vi "Populate Variant Database.vi"(8 "Error In":errorcluster, 10 "Data":string) -> (0 "Error Out":errorcluster, 1 "Variant DB":variant)   [LabVIEW 2017, in "Configit.lvlib"]
uses:
  Configit.lvlib
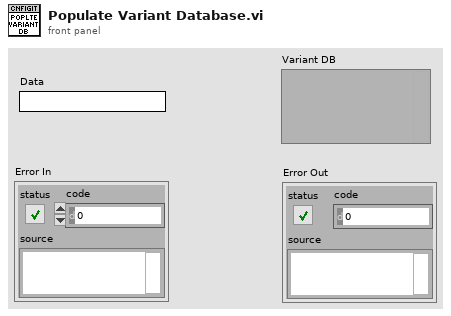
[diagram p1: front panel]
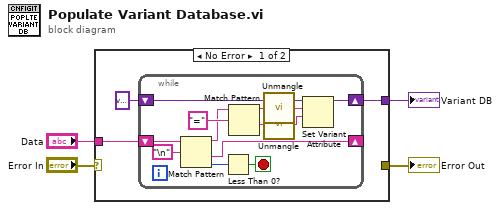
[diagram p0: block diagram]
diagram:
  n1 = case shown="No Error" "Error In" {
    selector: "Error In" -> [_ w21]
    tunnel: "Data" -> [w6 _]
    tunnel: [w5 _] -> w3
    tunnel: [_ w21] -> w1
    frame No Error {
      n2 = while {
        shift-right: [w16] -> w5
        shift-left: variant ("variant") -> [w17]
        shift-right: [w11] -> _
        shift-left: w6 -> [w9]
        stop <- w19 stop-if-true
        n3 = Match Pattern(string=w9, regular expression="\n") -> (before substring=w12:string, after substring=w11:string, offset past match=w8:i32)  [unwired: 1 in, 1 out]
        n4 = Less Than 0?(x=w8) -> (x < 0?=w19:bool)
        n5 = Match Pattern(string=w12, regular expression="=") -> (before substring=w15:string, after substring=w14:string)  [unwired: 1 in, 2 out]
        n6 = call "Unmangle.vi"("String In"=w15) -> ("String Out"=w10:string)
        n7 = call "Unmangle.vi"("String In"=w14) -> ("String Out"=w13:string)
        n8 = Set Variant Attribute(Variant=w17, name=w10, value=w13) -> (Variant out=w16:variant)  [unwired: 1 in, 2 out]
      }
    }
    frame Error {
    }
  }
  "Error Out" <- w1
  "Variant DB" <- w3
